vi "IPS Read Magnet Field.vi"(4 "Error In":errorcluster, 7 "VISA resource name":refnum<visa-resource-name>="COM3") -> (0 "Error Out":errorcluster, 1 "Persistent FIeld (T)":dbl, 2 "read buffer":string, 3 "VISA resource name":refnum<visa-resource-name>="GPIB1::25::INSTR")   [LabVIEW 2016, in "IPS-120.lvlib"]
uses:
  IPS-120.lvlib
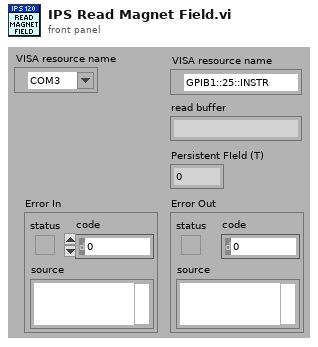
[diagram p1: front panel]
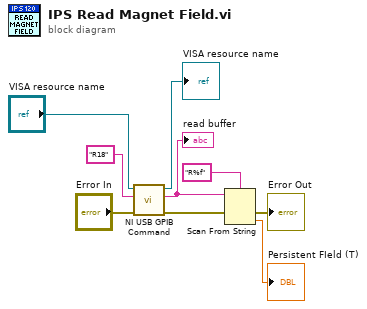
[diagram p0: block diagram]
diagram:
  n1 = call "NI USB GPIB Command.vi"("Error In"="Error In", "write buffer"="R18" ("String to Send"), "VISA resource name"="VISA resource name") -> ("Error Out"=w3:errorcluster, "read buffer"=w1:string, "VISA resource name out"=→"VISA resource name":refnum<visa-resource-name>)  [unwired: 6 in]
  "read buffer" <- w1
  n2 = Scan From String(format string="R%f", input string=w1, error in=w3) -> (error out=→"Error Out":errorcluster, output 1=→"Persistent FIeld (T)":dbl)  [unwired: 1 in, 3 out]
